vi "GetOutputShapeDim.vi"(8 "error in (no error)":errorcluster, 9 "dimIndex":i32, 10 "outputIndex":i32, 11 "session id in":i32) -> (0 "error out":errorcluster, 2 "OutputShapeDim":i64, 3 "session id out":i32)   [LabVIEW 2017, in "libonnx_wrapper.lvlib"]
doc: "/**\n * @brief Получить значение конкретной размерности выходного тензора\n * \n * Возвращает размер тензора по указанному измерению.\n * Например, для shape [1, 3, 224, 224]:\n * - dimIndex=0 вернёт 1 (батч)\n * - dimIndex=1 вернёт 3 (каналы)\n * - dimIndex=2 вернёт 224 (высота)\n * - dimIndex=3 вернёт 224 (ширина)\n * \n * @param sessionId [IN] ID сессии\n * @param outputIndex [IN] Индекс входа (0-based)\n * @param dimIndex [IN] Индекс размерности (0-based, от 0 до GetInputShapeDimCount-1)\n * \n * @return int64: Значение размерности (положительное число)\n * @return int64: -1 если сессия не найдена или индексы неверны\n */\nint64_t GetOutputShapeDim(int sessionId, int outputIndex, int dimIndex);"
uses:
  libonnx_wrapper.lvlib
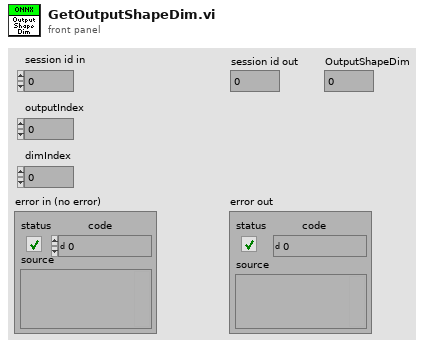
[diagram p1: front panel]
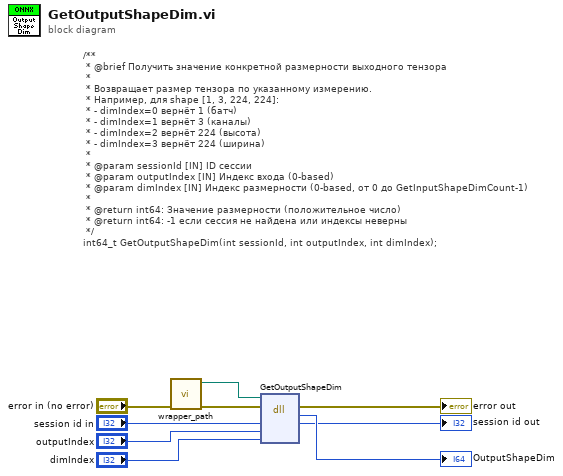
[diagram p0: block diagram]
diagram:
  # "/**\n * @brief Получить значение конкретной размерности выходного тензора\n * \n * Возвращает размер тензора по указанному измерению.\n * Например, для shape [1, 3, 224, 224]:\n * - dimIndex=0 вернёт 1 (батч)\n * - dimIndex=1 вернёт 3 (каналы)\n * - dimIndex=2 вернёт 224 (высота)\n * - dimIndex=3 вернёт 224 (ширина)\n * \n * @param sessionId [IN] ID сессии\n * @param outputIndex [IN] Индекс входа (0-based)\n * @param dimIndex [IN] Индекс размерности (0-based, от 0 до GetInputShapeDimCount-1)\n * \n * @return int64: Значение размерности (положительное число)\n * @return int64: -1 если сессия не найдена или индексы неверны\n */\nint64_t GetOutputShapeDim(int sessionId, int outputIndex, int dimIndex);"
  n1 = call "wrapper_path.vi"("error in (no error)"="error in (no error)") -> ("error out"=w3:errorcluster, "wrapper path"=w6:path)  [unwired: 9 in]
  n2 = dll-call lib="home/ivan/LabVIEWData/ONNX/Test/libonnx_wrapper/unix64/libonnx_wrapper.so" fn="GetOutputShapeDim"(path in=w6, error in=w3, "sessionId"="session id in", "outputIndex"="outputIndex", "dimIndex"="dimIndex") -> (error out=→"error out":errorcluster, "OutputShapeDim"=→"OutputShapeDim":i64, "sessionId"=→"session id out":i32)  [unwired: 3 in, 1 out]
